vi "Get Capacity Limits.vi"(4 "error in (no error)":errorcluster, 7 "VISA resource name":refnum<visa-resource-name>) -> (0 "error out":errorcluster, 1 "Maximum cooling capacity(out)":i8 min=-100 max=0, 2 "Maximum heating capacity(out)":u8=100 max=100, 3 "VISA resource name out":refnum<visa-resource-name>)   [LabVIEW 2018, in "JULABO DeviceDriver.lvlib"]
doc: "This VI returns the maximum allowed heating and cooling capacity in percent. 100 % corresponds to the technical specification of the equipment."
uses:
  JULABO DeviceDriver.lvlib
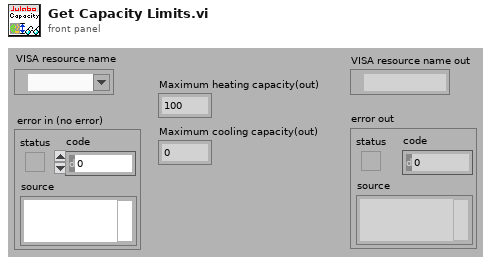
[diagram p1: front panel]
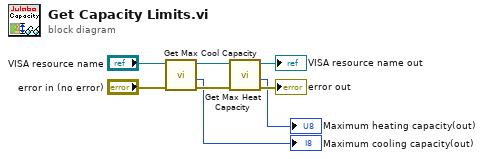
[diagram p0: block diagram]
diagram:
  n1 = call "Get Max Cool Capacity.vi"("error in (no error)"="error in (no error)", "VISA resource name"="VISA resource name") -> ("error out"=w5:errorcluster, "CoolMax (out)"=→"Maximum cooling capacity(out)":i8, "VISA resource name out"=w6:refnum<visa-resource-name>)  [unwired: 7 in]
  n2 = call "Get Max Heat Capacity.vi"("error in (no error)"=w5, "VISA resource name"=w6) -> ("error out"=→"error out":errorcluster, "HeatMax (out)"=→"Maximum heating capacity(out)":i8, "VISA resource name out"=→"VISA resource name out":refnum<visa-resource-name>)  [unwired: 7 in]
